vi "BIN-PAQ-day-GetFolderLocations.vi"(8 "error in (no error)":errorcluster, 9 "Time-End":timestamp, 11 "Time-Start":timestamp) -> (0 "error out":errorcluster, 1 "Overlap?":bool, 3 "Folders":string[](array[string]))   [LabVIEW 2020, in "Sgraph_lib_V1.lvlib" / "Gviewer.lvclass"]
doc: "Find the folders where the historian files are located for the 'per day' pace"
uses:
  Gview/Gviewer.lvclass
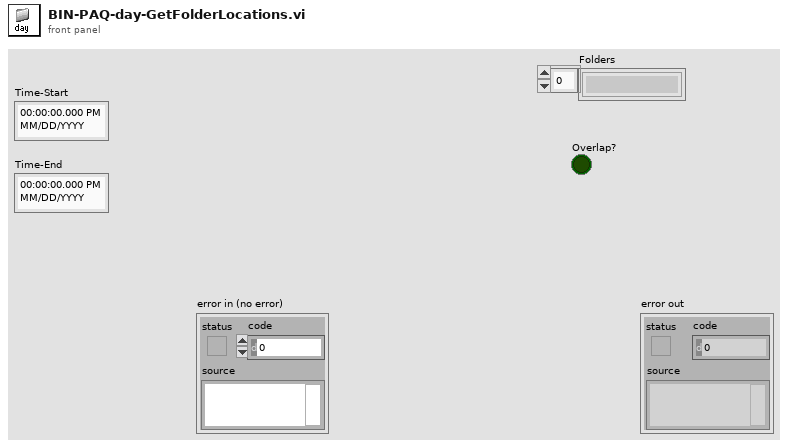
[diagram p1: front panel]
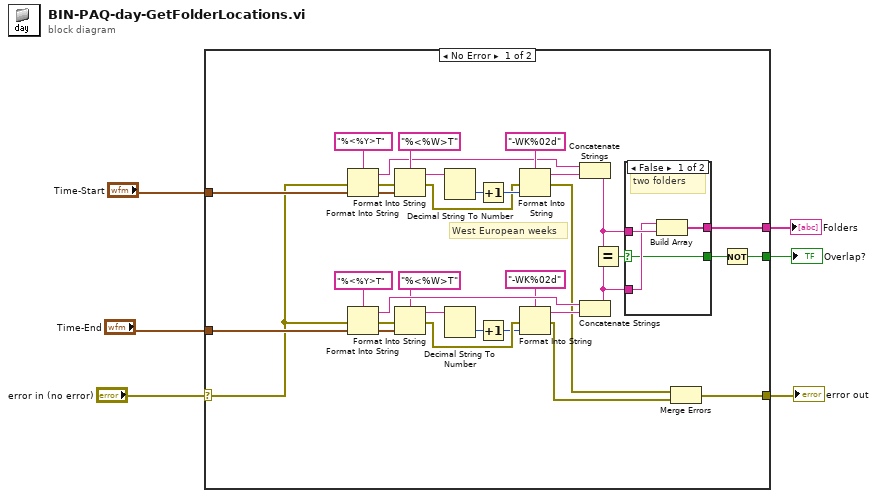
[diagram p0: block diagram]
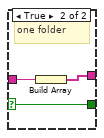
[diagram p2: hidden frame]
diagram:
  n1 = case shown="No Error" "error in (no error)" {
    selector: "error in (no error)" -> [w13 w46]
    tunnel: "Time-Start" -> [w15 _]
    tunnel: "Time-End" -> [w14 _]
    tunnel: [w10 w46] -> w3
    tunnel: [w9 _] -> w2
    tunnel: [w7 _] -> w1
    frame No Error {
      # "West European weeks"
      n2 = Format Into String(format string="%<%Y>T", error in=w13, w15) -> (resulting string=w29:string, error out=w36:errorcluster)  [unwired: 1 in]
      n3 = Format Into String(format string="%<%Y>T", error in=w13, w14) -> (resulting string=w28:string, error out=w21:errorcluster)  [unwired: 1 in]
      n4 = Format Into String(format string="%<%W>T", error in=w36, w15) -> (resulting string=w35:string, error out=w31:errorcluster)  [unwired: 1 in]
      n5 = Format Into String(format string="%<%W>T", error in=w21, w14) -> (resulting string=w22:string, error out=w26:errorcluster)  [unwired: 1 in]
      n6 = Decimal String To Number(string=w35) -> (number=w34:i32)  [unwired: 2 in, 1 out]
      n7 = Decimal String To Number(string=w22) -> (number=w23:i32)  [unwired: 2 in, 1 out]
      n8 = Increment(x=w34) -> (x+1=w33:i32)
      n9 = Increment(x=w23) -> (x+1=w24:i32)
      n10 = Format Into String(format string="-WK%02d", error in=w31, w33) -> (resulting string=w30:string, error out=w12:errorcluster)  [unwired: 1 in]
      n11 = Format Into String(format string="-WK%02d", error in=w26, w24) -> (resulting string=w27:string, error out=w11:errorcluster)  [unwired: 1 in]
      n12 = Concatenate Strings(w29, w30) -> (w17:string)
      n13 = Concatenate Strings(w28, w27) -> (w16:string)
      n14 = Equal?(x=w17, y=w16) -> (x = y?=w18:bool)
      n15 = case shown="False" w18 {
        selector: w18 -> [w39 w43]
        tunnel: w17 -> [w42 w45]
        tunnel: [w40 w44] -> w9
        tunnel: w16 -> [w41 _]
        tunnel: [w39 w43] -> w8
        frame False {
          # "two folders"
          n16 = Build Array(w41, w42) -> (w40:string[])
        }
        frame True {
          # "one folder"
          n17 = Build Array(w45) -> (w44:string[])
        }
      }
      n18 = Merge Errors(w12, w11) -> (w10:errorcluster)
      n19 = Not(x=w8) -> (.not. x?=w7:bool)
    }
    frame Error {
    }
  }
  "error out" <- w3
  "Folders" <- w2
  "Overlap?" <- w1
